vi "Read Row Data.vi"(7 "Section Name":string, 8 "error in (no error)":errorcluster, 9 "Col Header Val":string, 10 "Col Header Name":string, 11 "Config Data":T1(array[cluster])) -> (0 "error out":errorcluster, 1 "Column Data":string[](array[string]), 3 "Config Data dup":T1(array[cluster]), 4 "Key Find?":bool)   [LabVIEW 2020, in "GUCalibration2.lvlib"]
uses:
  GUCalibration2.lvlib
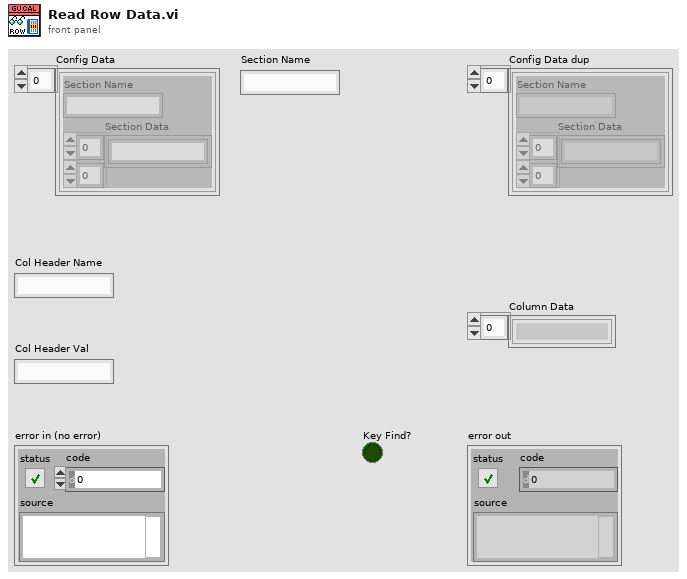
[diagram p1: front panel]
types:
  T1 = cluster{"Section Name":string, "Section Data":string[][]}[]
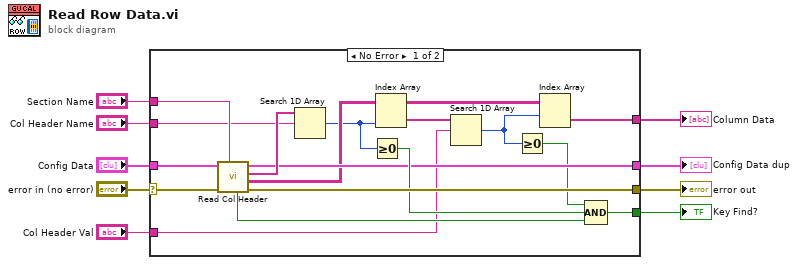
[diagram p0: block diagram]
diagram:
  n1 = case shown="No Error" "error in (no error)" {
    selector: "error in (no error)" -> [w24 w28]
    tunnel: "Section Name" -> [w25 _]
    tunnel: "Config Data" -> [w26 w27]
    tunnel: [w21 w28] -> w6
    tunnel: [w17 w27] -> w5
    tunnel: [w18 _] -> w4
    tunnel: [w10 _] -> w3
    tunnel: "Col Header Name" -> [w22 _]
    tunnel: "Col Header Val" -> [w15 _]
    frame No Error {
      n2 = call "Read Col Header.vi"("Section Name"=w25, "error in (no error)"=w24, "Config Data"=w26) -> ("error out"=w21:errorcluster, "Data"=w13:string[][], "Column Header"=w23:string[], "Config Data dup"=w17:T1, "Section Find?"=w19:bool)  [unwired: 4 in]
      n3 = Search 1D Array(1D array=w23, element=w22) -> (index of element=w11:i32)  [unwired: 1 in]
      n4 = Greater Or Equal To 0?(x=w11) -> (x >= 0?=w20:bool)
      n5 = Index Array(array=w13, index (col)=w11) -> (element=w16:string[])  [unwired: 1 in]
      n6 = Search 1D Array(1D array=w16, element=w15) -> (index of element=w12:i32)  [unwired: 1 in]
      n7 = Greater Or Equal To 0?(x=w12) -> (x >= 0?=w14:bool)
      n8 = Index Array(array=w13, index (row)=w12) -> (element=w10:string[])  [unwired: 1 in]
      n9 = Compound Arithmetic op=AND(w14, w20, w19) -> (w18:bool)
    }
    frame Error {
    }
  }
  "error out" <- w6
  "Column Data" <- w3
  "Config Data dup" <- w5
  "Key Find?" <- w4
